vi "System Spec Widget.vi"(8 "Error In":errorcluster) -> (0 "Error Out":errorcluster, 3 "New System Spec Widget":refnum<class "System Spec Widget.lvclass">)   [LabVIEW 2013, in "System Spec Widget.lvclass"]
doc: "Copyright (c) 2016 Sze Howe Koh\nThis code is licensed under the MIT license"
uses:
  System Spec Widget.lvclass
  src/LabVIEW/LQ Core/Qt/AlignmentFlag.ctl
  System Spec Widget.lvclass/System Spec Widget.ctl
  src/LabVIEW/Qt Widgets/QSpinBox/setSuffix.vi
  src/LabVIEW/Qt Widgets/QSpinBox/setMaximum.vi
  src/LabVIEW/Qt Widgets/QSpinBox/setMinimum.vi
  src/LabVIEW/Qt Widgets/QSpinBox/setValue.vi
  src/LabVIEW/Qt Widgets/QFormLayout/setLabelAlignment.vi
  src/LabVIEW/Qt Widgets/QWidget/QWidget.lvclass
  src/LabVIEW/Qt Widgets/QGroupBox/QGroupBox.lvclass
  src/LabVIEW/Qt Widgets/QSpinBox/QSpinBox.lvclass
  src/LabVIEW/Qt Widgets/QFormLayout/QFormLayout.lvclass
  src/LabVIEW/LQ Core/Qt/Qt.lvlib
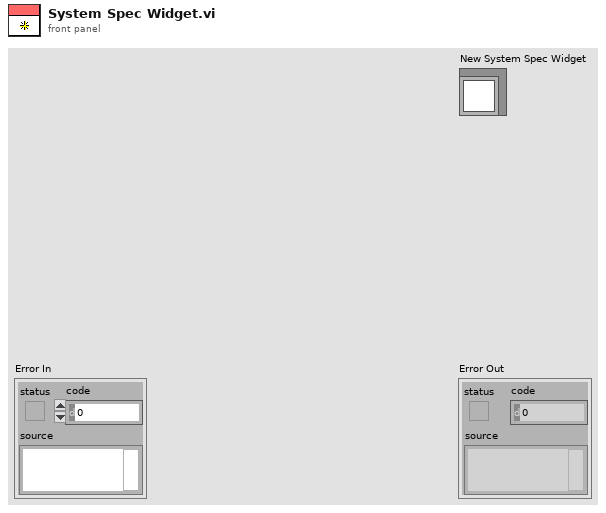
[diagram p1: front panel]
types:
  T1 = typedef "Qt.lvlib/AlignmentFlag.ctl" = i32
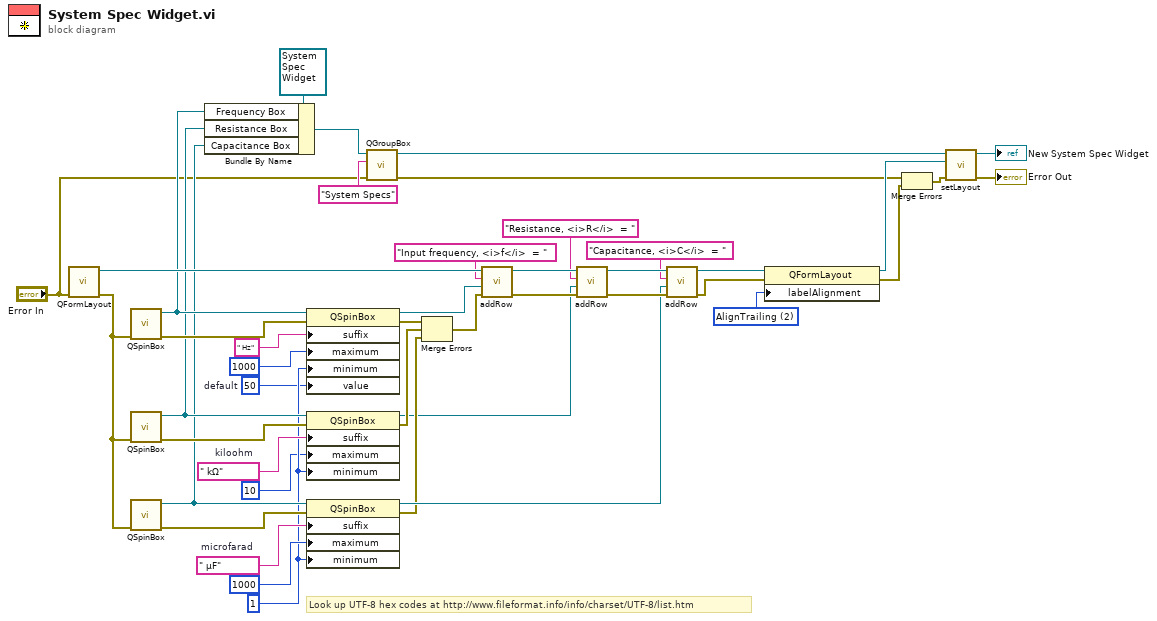
[diagram p0: block diagram]
diagram:
  w1 = 50  # default
  w4 = 1 ("maximum")
  w30 = T1 2 items=["AlignLeading"=1, "AlignTrailing"=2, "AlignHCenter"=4, "AlignJustify"=8, "AlignAbsolute"=16, "AlignHorizontal_Mask"=31, "AlignTop"=32, "AlignBottom"=64, "AlignVCenter"=128, "AlignBaseline"=256, "AlignVertical_Mask"=480, "AlignCenter"=132] ("labelAlignment")
  w23 = " μF"  # microfarad
  w22 = " kΩ"  # kiloohm
  # "Look up UTF-8 hex codes at http://www.fileformat.info/info/charset/UTF-8/list.htm"
  n1 = call "QFormLayout.vi"("Error In"="Error In") -> ("Error Out"=w8:errorcluster, "New QFormLayout"=w38:refnum<class "QFormLayout.lvclass">)  [unwired: 9 in]
  n2 = call "QSpinBox.vi"("Error In"=w8) -> ("Error Out"=w40:errorcluster, "New QSpinBox"=w11:refnum<class "QSpinBox.lvclass">)  [unwired: 9 in]
  n3 = call "QSpinBox.vi"("Error In"=w8) -> ("Error Out"=w29:errorcluster, "New QSpinBox"=w10:refnum<class "QSpinBox.lvclass">)  [unwired: 9 in]
  n4 = call "QSpinBox.vi"("Error In"=w8) -> ("Error Out"=w28:errorcluster, "New QSpinBox"=w9:refnum<class "QSpinBox.lvclass">)  [unwired: 9 in]
  n5 = Bundle By Name(cluster=refnum<class "System Spec Widget.lvclass"> refnum ("System Spec Widget"), "Frequency Box"=w11, "Resistance Box"=w10, "Capacitance Box"=w9) -> (w12:refnum<class "System Spec Widget.lvclass">)
  n6 = property class="QSpinBox"(reference=w11, error in=w40, "suffix"=" Hz" ("text"), "maximum"=1000, "minimum"=w4, "value"=w1) -> (reference out=w14:refnum<class "QSpinBox.lvclass">, error out=w15:errorcluster)
  n7 = property class="QSpinBox"(reference=w10, error in=w29, "suffix"=w22, "maximum"=10, "minimum"=w4) -> (reference out=w16:refnum<class "QSpinBox.lvclass">, error out=w17:errorcluster)
  n8 = property class="QSpinBox"(reference=w9, error in=w28, "suffix"=w23, "maximum"=1000, "minimum"=w4) -> (reference out=w19:refnum<class "QSpinBox.lvclass">, error out=w18:errorcluster)
  n9 = call "QGroupBox.vi"("Error In"="Error In", "title"="System Specs", "Post-Bundled Subclass"=w12) -> ("Error Out"=w21:errorcluster, "New QGroupBox"=w20:refnum<class "System Spec Widget.lvclass">)  [unwired: 7 in]
  n10 = Merge Errors(w15, w17, w18) -> (w25:errorcluster)
  n11 = call "addRow.vi"("Error In"=w25, "field"=w14, "labelText"="Input frequency, <i>f</i>  = " ("text"), "QFormLayout In"=w38) -> ("Error Out"=w24:errorcluster, "QFormLayout Out"=w37:refnum<class "QFormLayout.lvclass">)  [unwired: 6 in]
  n12 = call "addRow.vi"("Error In"=w24, "field"=w16, "labelText"="Resistance, <i>R</i>  = " ("text"), "QFormLayout In"=w37) -> ("Error Out"=w44:errorcluster, "QFormLayout Out"=w36:refnum<class "QFormLayout.lvclass">)  [unwired: 6 in]
  n13 = call "addRow.vi"("Error In"=w44, "field"=w19, "labelText"="Capacitance, <i>C</i>  = " ("text"), "QFormLayout In"=w36) -> ("Error Out"=w27:errorcluster, "QFormLayout Out"=w32:refnum<class "QFormLayout.lvclass">)  [unwired: 6 in]
  n14 = property class="QFormLayout"(reference=w32, error in=w27, "labelAlignment"=w30) -> (reference out=w31:refnum<class "QFormLayout.lvclass">, error out=w7:errorcluster)
  n15 = Merge Errors(w21, w7) -> (w6:errorcluster)
  n16 = call "setLayout.vi"("Error In"=w6, "layout"=w31, "QWidget In"=w20) -> ("Error Out"=→"Error Out":errorcluster, "QWidget Out"=→"New System Spec Widget":refnum<class "System Spec Widget.lvclass">)  [unwired: 7 in]
